vi "SolarThermal.vi"(5 "Day of Year":u32, 6 "Unique Object Identifier":string, 7 "Day Time":u32, 8 "Error In":errorcluster, 10 "Energy flow IN":T5, 11 "DataFlowIN":T4) -> (0 "Error Out":errorcluster, 2 "Energy flow OUT":T5, 3 "DataFlowOUT":T4)   [LabVIEW 2017]
uses:
  classes/DataCollector.lvclass
  classes/DataHandler.lvclass
  classes/SimulationParameter.lvclass
panel:
  out "Simulation Parameter":T1
  in  "Operating Parameter":T2
  out "Control Parameter":T3
  out "List of Fieldelements":string[](array[string])
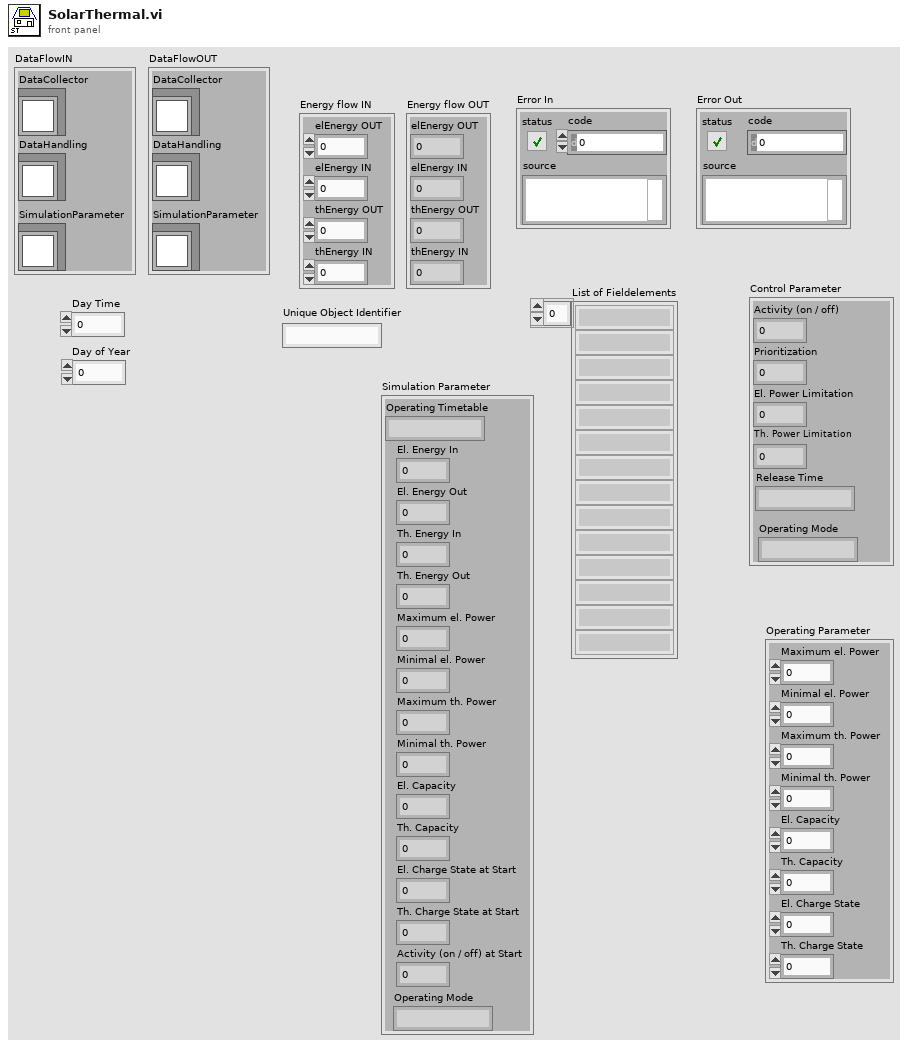
[diagram p1: front panel]
types:
  T1 = cluster{"Operating Timetable":string, "El. Energy In":dbl, "El. Energy Out":dbl, "Th. Energy In":dbl, "Th. Energy Out":dbl, "Maximum el. Power":dbl, "Minimal el. Power":dbl, "Maximum th. Power":dbl, "Minimal th. Power":dbl, "El. Capacity":dbl, "Th. Capacity":dbl, "El. Charge State at Start":dbl, "Th. Charge State at Start":dbl, "Activity (on / off) at Start":i64, "Operating Mode":string}
  T2 = cluster{"Maximum el. Power":dbl, "Minimal el. Power":dbl, "Maximum th. Power":dbl, "Minimal th. Power":dbl, "El. Capacity":dbl, "Th. Capacity":dbl, "El. Charge State":dbl, "Th. Charge State":dbl}
  T3 = cluster{"Activity (on / off)":i64, "Prioritization":i64, "El. Power Limitation":dbl, "Th. Power Limitation":dbl, "Release Time":string, "Operating Mode":string}
  T4 = cluster{"DataCollector":refnum<class "DataCollector.lvclass">, "DataHandling":refnum<class "DataHandler.lvclass">, "SimulationParameter":refnum<class "SimulationParameter.lvclass">}
  T5 = cluster{"elEnergy OUT":dbl, "elEnergy IN":dbl, "thEnergy OUT":dbl, "thEnergy IN":dbl}
  T6 = cluster{"elEnergy OUT":dbl, "thEnergy OUT":dbl, "thEnergy IN":dbl, "thEnergy IN":dbl}
  T7 = cluster{"Day Time":u32, "Day of Year":u32, cluster{"elEnergy OUT":dbl, "thEnergy OUT":dbl, "thEnergy IN":dbl, "thEnergy IN":dbl}, "Operating Parameter":cluster{"Maximum el. Power":dbl, "Minimal el. Power":dbl, "Maximum th. Power":dbl, "Minimal th. Power":dbl, "El. Capacity":dbl, "Th. Capacity":dbl, "El. Charge State":dbl, "Th. Charge State":dbl}, "Control Parameter":cluster{"Activity (on / off)":i64, "Prioritization":i64, "El. Power Limitation":dbl, "Th. Power Limitation":dbl, "Release Time":string, "Operating Mode":string}}
  T8 = cluster{"elEnergy OUT":dbl, "thEnergy OUT":dbl, "Power Out":dbl, "thEnergy IN":dbl}
  T9 = cluster{"Day Time":u32, "Day of Year":u32, cluster{"elEnergy OUT":dbl, "thEnergy OUT":dbl, "Power Out":dbl, "thEnergy IN":dbl}, "Operating Parameter":cluster{"Maximum el. Power":dbl, "Minimal el. Power":dbl, "Maximum th. Power":dbl, "Minimal th. Power":dbl, "El. Capacity":dbl, "Th. Capacity":dbl, "El. Charge State":dbl, "Th. Charge State":dbl}, "Control Parameter":cluster{"Activity (on / off)":i64, "Prioritization":i64, "El. Power Limitation":dbl, "Th. Power Limitation":dbl, "Release Time":string, "Operating Mode":string}}
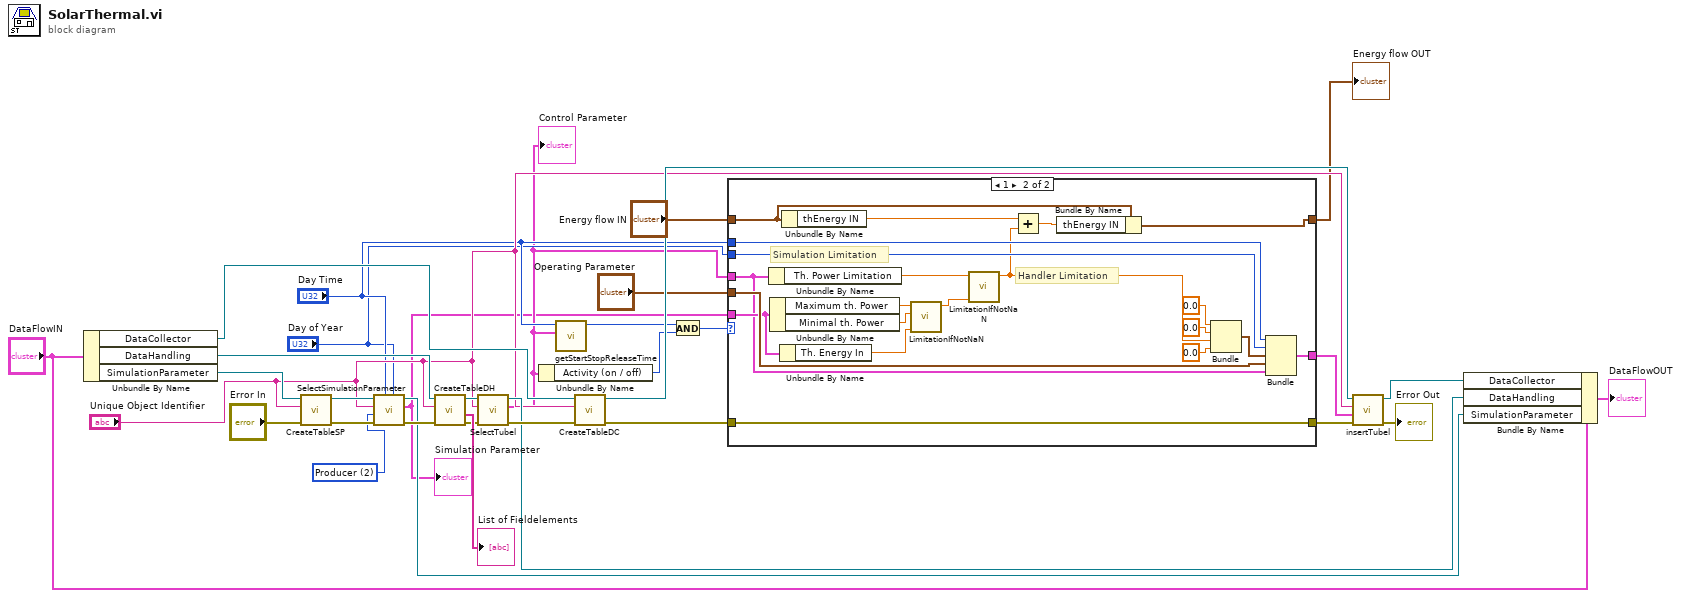
[diagram p0: block diagram]
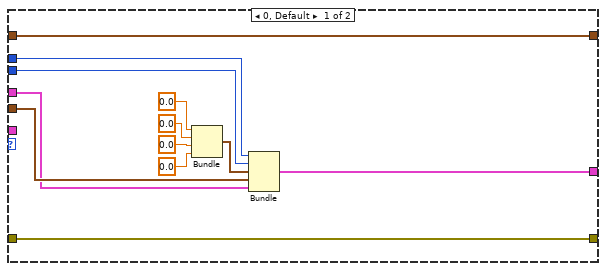
[diagram p2: hidden frame]
diagram:
  w1 = u16 2 items=["External Network", "Consumer", "Producer", "Sorage"] ("Type of Simulation")
  n1 = Unbundle By Name("DataFlowIN") -> ("DataCollector"=w33:refnum<class "DataCollector.lvclass">, "DataHandling"=w23:refnum<class "DataHandler.lvclass">, "SimulationParameter"=w17:refnum<class "SimulationParameter.lvclass">)
  n2 = call-dynamic "CreateTableSP.vi"("error in (no error)"="Error In", "Name of Table"="Unique Object Identifier", "SimulationParameter in"=w17) -> ("error out"=w21:errorcluster, "SimulationParameter out"=w20:refnum<class "SimulationParameter.lvclass">)  [unwired: 5 in, 2 out]
  n3 = call-dynamic "SelectSimulationParameter.vi"("Day of Year"="Day of Year", "Day Time"="Day Time", "error in (no error)"=w21, "Type of Simulation"=w1, "Unique Object Identifier"="Unique Object Identifier", "SimulationParameter in"=w20) -> ("error out"=w19:errorcluster, "Cluster"=w3:T1, "SimulationParameter out"=w15:refnum<class "SimulationParameter.lvclass">)  [unwired: 3 in]
  "Simulation Parameter" <- w3
  n4 = call-dynamic "CreateTableDH.vi"("error in (no error)"=w19, "Name of Table"="Unique Object Identifier", "DataHandler in"=w23) -> ("error out"=w25:errorcluster, "List of Fieldelements"=→"List of Fieldelements":string[], "DataHandler out"=w26:refnum<class "DataHandler.lvclass">)  [unwired: 5 in, 1 out]
  n5 = call-dynamic "SelectTubel.vi"("error in (no error)"=w25, "Unique Object Identifier"="Unique Object Identifier", "DataHandler in"=w26) -> ("error out"=w24:errorcluster, "Control Parameter"=w4:T3, "DataHandler out"=w22:refnum<class "DataHandler.lvclass">)  [unwired: 5 in, 1 out]
  "Control Parameter" <- w4
  n6 = Unbundle By Name(w4) -> ("Activity (on / off)"=w14:i64)
  n7 = call "getStartStopReleaseTime.vi"("Control Parameter"=w4, "Day Time"="Day Time") -> ("Activity (on / off)"=w13:i64)  [unwired: 9 in]
  n8 = call "CreateTableDC.vi"("error in (no error)"=w24, "Name of Table"="Unique Object Identifier", "DataCollector in"=w33) -> ("error out"=w11:errorcluster, "DataCollector out"=w32:refnum<class "DataCollector.lvclass">)  [unwired: 7 in]
  n9 = And(x=w13, y=w14) -> (x .and. y?=w12:i64)
  n10 = case shown="1" w12 {
    tunnel: w11 -> [w44 w52]
    tunnel: [w44 w52] -> w10
    tunnel: "Day Time" -> [w37 w66]
    tunnel: "Day of Year" -> [w36 w65]
    tunnel: "Operating Parameter" -> [w39 w64]
    tunnel: "Energy flow IN" -> [w45 w62]
    tunnel: [w45 w60] -> w8
    tunnel: w3 -> [_ w61]
    tunnel: w4 -> [w34 w50]
    tunnel: [w35 w51] -> w2
    frame 0, Default {
      n11 = Bundle("elEnergy OUT"=0.0, "thEnergy OUT"=0.0, "thEnergy IN"=0.0, "thEnergy IN"=0.0) -> (w38:T6)  [unwired: 1 in]
      n12 = Bundle("Day Time"=w37, "Day of Year"=w36, w38, "Operating Parameter"=w39, "Control Parameter"=w34) -> (w35:T7)  [unwired: 1 in]
    }
    frame 1 {
      # "Simulation Limitation"
      # "Handler Limitation"
      n13 = Unbundle By Name(w50) -> ("Th. Power Limitation"=w56:dbl)
      n14 = Unbundle By Name(w61) -> ("Maximum th. Power"=w59:dbl, "Minimal th. Power"=w58:dbl)
      n15 = Unbundle By Name(w61) -> ("Th. Energy In"=w57:dbl)
      n16 = Unbundle By Name(w62) -> ("thEnergy IN"=w63:dbl)
      n17 = call "LimitationIfNotNaN.vi"("x"=w57, "Minimal Power"=w58, "Maximum Power"=w59) -> ("Power Out"=w55:dbl)  [unwired: 7 in, 1 out]
      n18 = call "LimitationIfNotNaN.vi"("x"=w55, "Maximum Power"=w56) -> ("Power Out"=w49:dbl)  [unwired: 8 in, 1 out]
      n19 = Add(x=w63, y=w49) -> (x+y=w54:dbl)
      n20 = Bundle By Name(cluster=w62, "thEnergy IN"=w54) -> (w60:T5)
      n21 = Bundle("elEnergy OUT"=0.0, "thEnergy OUT"=0.0, "Power Out"=w49, "thEnergy IN"=0.0) -> (w53:T8)  [unwired: 1 in]
      n22 = Bundle("Day Time"=w66, "Day of Year"=w65, w53, "Operating Parameter"=w64, "Control Parameter"=w50) -> (w51:T9)  [unwired: 1 in]
    }
  }
  "Energy flow OUT" <- w8
  n23 = call-dynamic "insertTubel.vi"("error in (no error)"=w10, "Data Cluster"=w2, "Name of Table"="Unique Object Identifier", "DataCollector in"=w32) -> ("error out"=→"Error Out":errorcluster, "DataCollector out"=w30:refnum<class "DataCollector.lvclass">)  [unwired: 6 in]
  n24 = Bundle By Name(cluster="DataFlowIN", "DataCollector"=w30, "DataHandling"=w22, "SimulationParameter"=w15) -> (→"DataFlowOUT":T4)
